vi "Adquisicion_6008.vi"() -> ()   [LabVIEW 2011]
uses:
  <vilib>/Utility/config.llb/Read Key (String).vi
  <vilib>/Utility/config.llb/Read Key (Double).vi
  <vilib>/Utility/config.llb/Write Key (String).vi
  <vilib>/Utility/config.llb/Write Key (Double).vi
  <vilib>/Utility/config.llb/NI_LVConfig.lvlib
  <vilib>/Analysis/NI_AALBase.lvlib
panel:
  out "Boolean 10":bool
  in  "Guardar":bool
  in  "Path2":bool
  in  "Datapath":bool
  in  "Path1":bool=TRUE
  in  "Tiempo":dbl
  in  "index 3":i32
  in  "index":i32
  out "reset3":bool
  out "reset2":bool
  out "reset":bool
  out "Time has Elapsed 2":bool caption="Time has Elapsed"
  out "Time has Elapsed":bool
  out "appended array":string[](array[string])
  in  "Tab Control 9":enum32{"Page 1", "Page 2", "Page 3"}(tab)
  in  "Tasa de Adquisicion":dbl=1000.0
  in  "CH8":string="CH8"
  in  "CH7":string="CH7"
  in  "CH6":string="CH6"
  in  "CH5":string="CH5"
  in  "CH4 2":string="CH4"
  in  "CH3":string="CH3"
  in  "CH2 2":string="CH2"
  in  "CH1":string="CH1"
  out "Voltaje":dbl
  out "Medida":dbl
  in  "m1":dbl
  in  "b1":dbl
  out "Voltaje":dbl
  in  "m2":dbl
  in  "b2":dbl
  out "Medida":dbl
  in  "m3":dbl
  in  "m4":dbl
  in  "b3":dbl
  in  "b4":dbl
  out "Voltaje":dbl
  out "Voltaje":dbl
  out "Medida":dbl
  out "Medida":dbl
  out "Medida":dbl
  in  "b5":dbl
  in  "m5":dbl
  out "Voltaje":dbl
  out "Medida":dbl
  in  "m6":dbl
  in  "b6":dbl
  out "Voltaje":dbl
  out "Medida":dbl
  in  "m7":dbl
  in  "b7":dbl
  out "Voltaje":dbl
  out "Voltaje":dbl
  in  "b8":dbl
  in  "m8":dbl
  out "Medida":dbl
  out "CH1":string
  out "CH2":string
  out "CH3":string
  out "CH4":string
  out "CH5":string
  out "CH6":string
  out "CH7":string
  out "CH8":string
  in  "Boolean":bool=TRUE
  in  "Boolean 2":bool=TRUE
  in  "Boolean 3":bool=TRUE
  in  "Boolean 4":bool=TRUE
  in  "Boolean 6":bool=TRUE
  in  "Boolean 5":bool=TRUE
  in  "Boolean 7":bool=TRUE
  in  "Boolean 8":bool=TRUE
  in  "Numero de Muestras":i32=1
  in  "file path":path=path "C:/Users/Zulueta/Documents/Pasantia/Mediciones"
  out "Tiempo":dbl caption="Elapsed Time (s)"
  in  "Iniciar":bool
  out "Boolean 9":bool
  in  "reset 2":bool caption="reset"
  out "q'":bool
  out "Tiempo":dbl caption="Elapsed Time (s)"
  in  "file path 2":path=path "C:/Users/Zulueta/Documents/Pasantia/Mediciones_Tiempo"
  out "Tiempo":dbl caption="Elapsed Time (s)"
  out "q2'":bool
  in  "?":bool
  in  "file path 3":path=path "C:/Users/Zulueta/Documents/Pasantia/Mediciones_Promedio"
  in  "Tiempo \nde adquisición":enum32{"Segundos", "Minutos", "Horas"}(tab) caption="Tiempo de adquisición"
  in  "?":dbl
  in  "?":dbl
  in  "?":dbl
  in  "stop":bool
  in  "Guardar Configuracion":bool
  out "Waveform Chart 10":dbl(graph)
  out "Waveform Chart 9":dbl(graph)
  out "Waveform Chart 8":dbl(graph)
  out "Waveform Chart 7":dbl(graph)
  out "Waveform Chart 6":dbl(graph)
  out "Waveform Chart 5":dbl(graph)
  out "Waveform Chart 4":dbl(graph)
  out "Waveform Chart 3":dbl(graph)
  out "CH1":string
  out "CH2":string
  out "CH3":string
  out "CH4":string
  out "CH5":string
  out "CH6":string
  out "CH7":string
  out "CH8":string
  in  "Boolean 18":bool=TRUE
  in  "Boolean 19":bool=TRUE
  in  "Boolean 20":bool=TRUE
  in  "Boolean 21":bool=TRUE
  in  "Boolean 22":bool=TRUE
  in  "Boolean 23":bool=TRUE
  in  "Boolean 24":bool=TRUE
  in  "Boolean 25":bool=TRUE
  out "Waveform Chart":cluster{dbl, dbl, dbl, dbl, dbl, dbl, dbl, dbl}(graph)
  out "Time":dbl
  # "On/Off"
  # "Pendiente"
  # "Medida"
  # "Offset"
  # "Voltaje"
  # "Aquirir muestras por solicitud"
  # "Adquirir muestras por tiempo definido"
  # "Adquirir promedio de cada canal en un tiempo T"
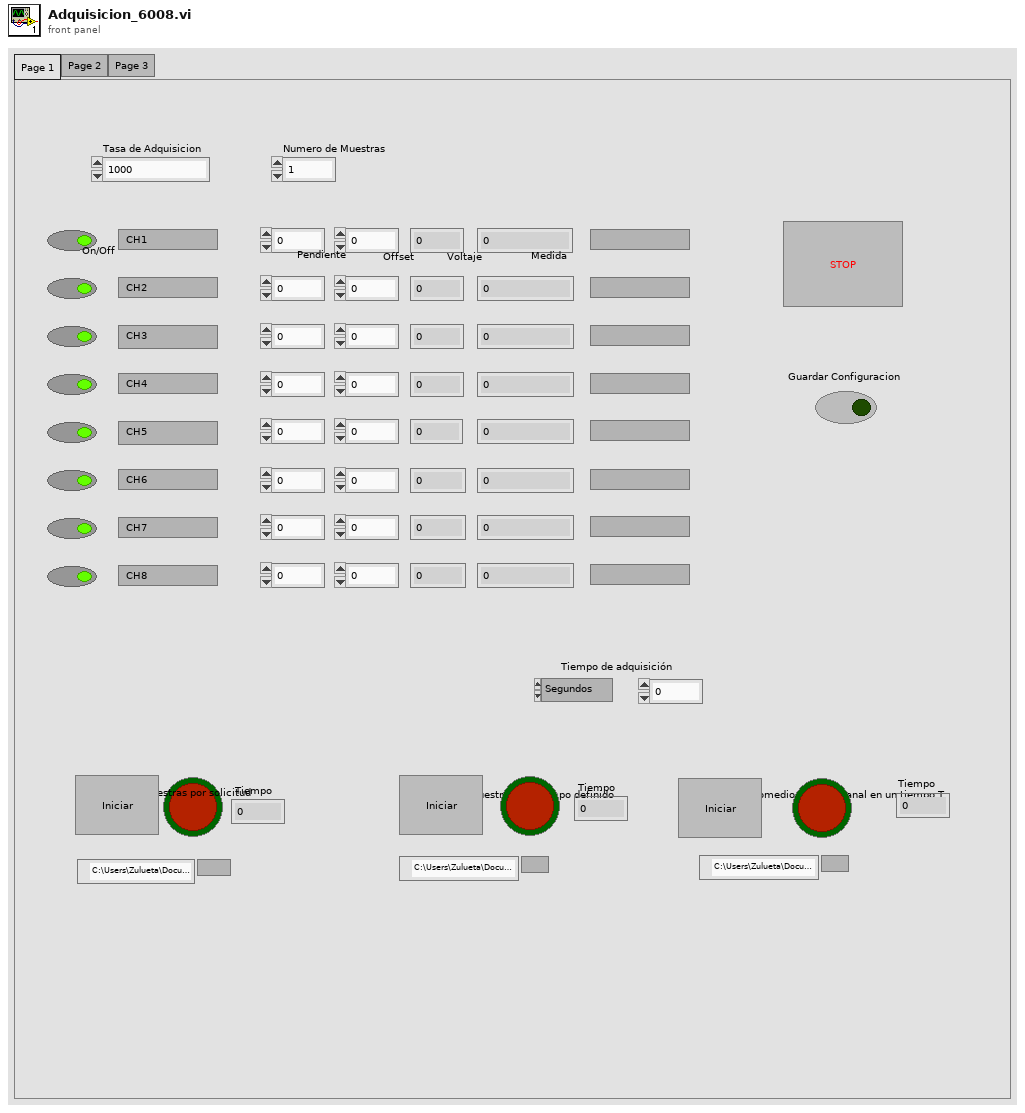
[diagram p1: front panel]
types:
  T1 = enum16{"big-endian, network order", "native, host order", "little-endian"}
  T2 = enum16{"open", "open or create", "create or replace", "create", "open (read-only)"}
  T3 = typedef "NI_LVConfig.lvlib/Config Data RefNum.ctl" = refnum<k1>
  T4 = cluster{"mean":dbl, "mean":dbl, "mean":dbl, "mean":dbl, "mean":dbl, "mean":dbl, "mean":dbl, "mean":dbl}
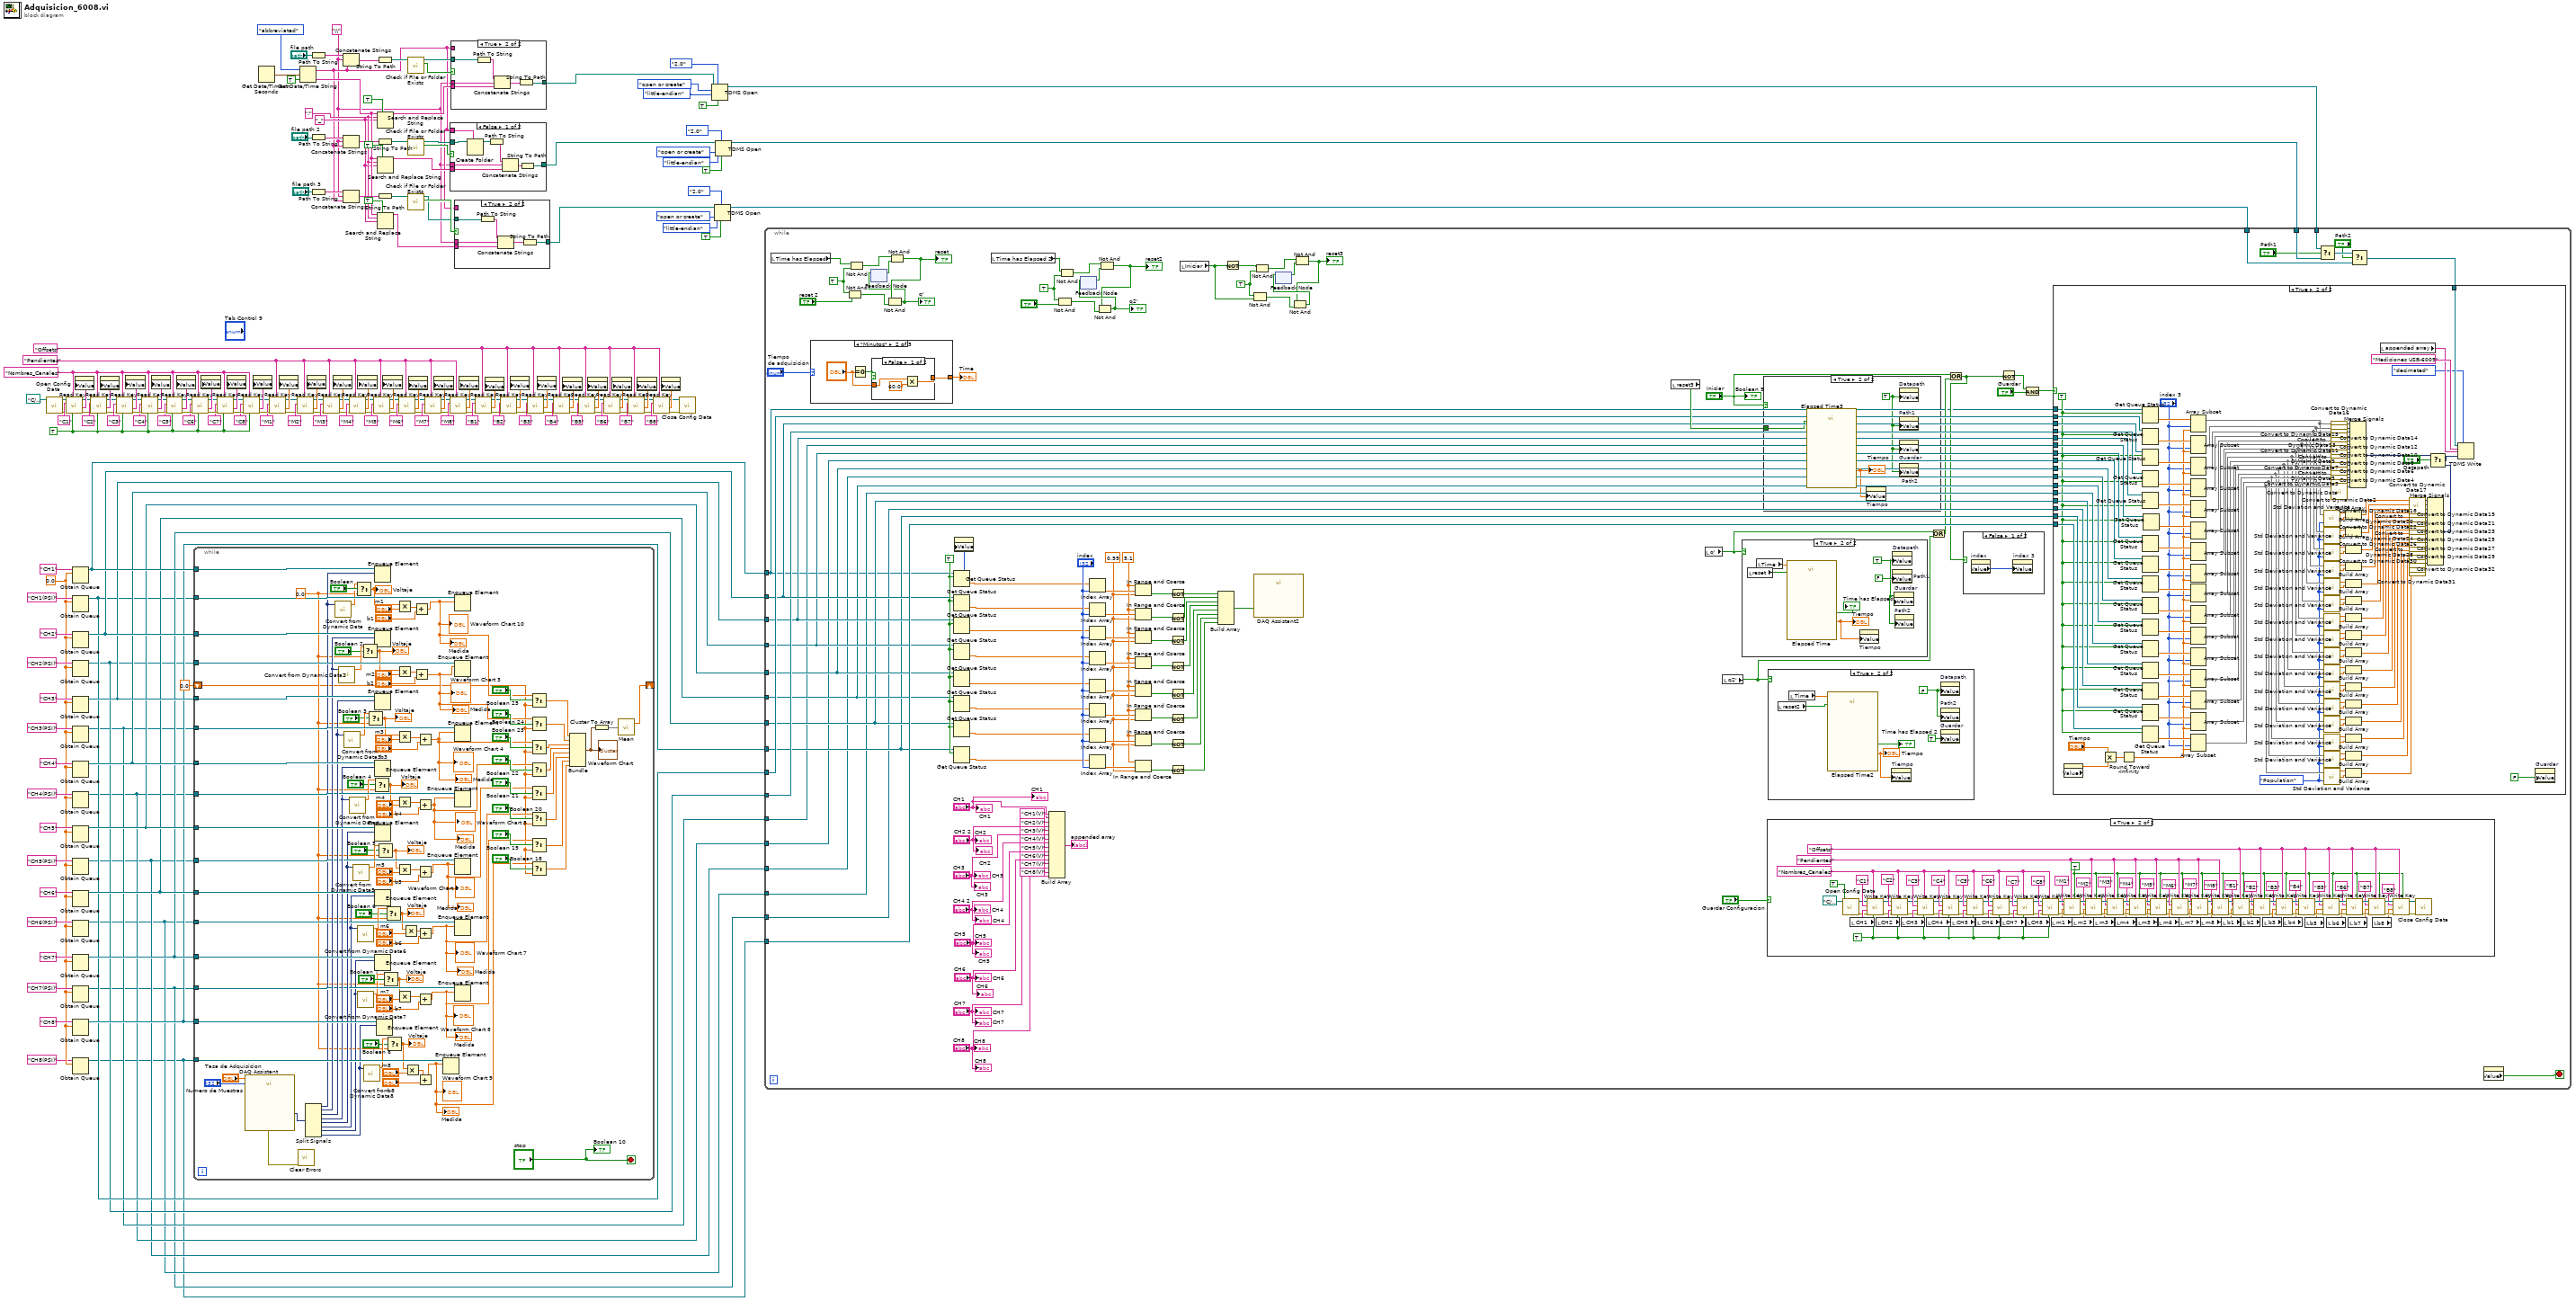
[diagram p0: block diagram]
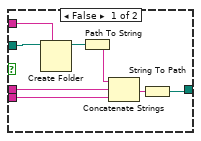
[diagram p2: hidden frame]
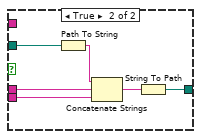
[diagram p3: hidden frame]
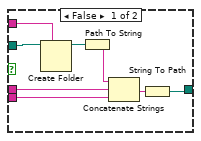
[diagram p4: hidden frame]
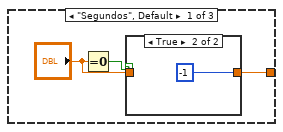
[diagram p11: hidden frame]
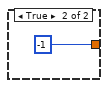
[diagram p13: hidden frame]
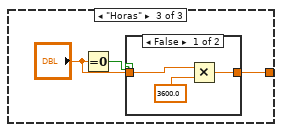
[diagram p14: hidden frame]
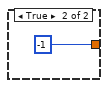
[diagram p15: hidden frame]
diagram:
  w25 = "_" ("replace string (\"\")")
  w26 = ":" ("search string")
  w9 = "\\" ("string")
  w71 = 0.0
  w88 = "Offsets" ("section")
  w121 = "Pendientes" ("section")
  w153 = TRUE ("read raw string? (F)")
  w154 = "Nombres_Canales" ("section")
  n1 = call <vilib>:"Open Config Data.vi"("configuration file path"=path "C:/Users/Zulueta/Documents/Pasantia/Configuracion") -> ("error out"=w183:errorcluster, "refnum"=w184:T3)  [unwired: 8 in, 1 out]
  n2 = call-poly <vilib>:"Read Key.vi"("read raw string? (F)"=w153, "section"=w154, "error in (no error)"=w183, "key"="C1", "refnum"=w184) -> ("error out"=w179:errorcluster, "value"=w186:string, "refnum out"=w180:T3)  [unwired: 3 in, 1 out]
  n3 = Obtain Queue(name (unnamed)="CH1", element data type=w71) -> (queue out=w69:refnum<queue>)  [unwired: 3 in, 2 out]
  n4 = Obtain Queue(name (unnamed)="CH1(PSI)", element data type=w71) -> (queue out=w59:refnum<queue>)  [unwired: 3 in, 2 out]
  n5 = Obtain Queue(name (unnamed)="CH2", element data type=w71) -> (queue out=w68:refnum<queue>)  [unwired: 3 in, 2 out]
  n6 = Obtain Queue(name (unnamed)="CH2(PSI)", element data type=w71) -> (queue out=w58:refnum<queue>)  [unwired: 3 in, 2 out]
  n7 = Obtain Queue(name (unnamed)="CH3", element data type=w71) -> (queue out=w67:refnum<queue>)  [unwired: 3 in, 2 out]
  n8 = Obtain Queue(name (unnamed)="CH3(PSI)", element data type=w71) -> (queue out=w57:refnum<queue>)  [unwired: 3 in, 2 out]
  n9 = Obtain Queue(name (unnamed)="CH4", element data type=w71) -> (queue out=w66:refnum<queue>)  [unwired: 3 in, 2 out]
  n10 = Obtain Queue(name (unnamed)="CH4(PSI)", element data type=w71) -> (queue out=w56:refnum<queue>)  [unwired: 3 in, 2 out]
  n11 = Obtain Queue(name (unnamed)="CH5", element data type=w71) -> (queue out=w65:refnum<queue>)  [unwired: 3 in, 2 out]
  n12 = Obtain Queue(name (unnamed)="CH5(PSI)", element data type=w71) -> (queue out=w55:refnum<queue>)  [unwired: 3 in, 2 out]
  n13 = Obtain Queue(name (unnamed)="CH6", element data type=w71) -> (queue out=w64:refnum<queue>)  [unwired: 3 in, 2 out]
  n14 = Obtain Queue(name (unnamed)="CH6(PSI)", element data type=w71) -> (queue out=w54:refnum<queue>)  [unwired: 3 in, 2 out]
  n15 = Obtain Queue(name (unnamed)="CH7", element data type=w71) -> (queue out=w63:refnum<queue>)  [unwired: 3 in, 2 out]
  n16 = Obtain Queue(name (unnamed)="CH7(PSI)", element data type=w71) -> (queue out=w53:refnum<queue>)  [unwired: 3 in, 2 out]
  n17 = Obtain Queue(name (unnamed)="CH8", element data type=w71) -> (queue out=w62:refnum<queue>)  [unwired: 3 in, 2 out]
  n18 = Obtain Queue(name (unnamed)="CH8(PSI)", element data type=w71) -> (queue out=w52:refnum<queue>)  [unwired: 3 in, 2 out]
  n19 = property on="CH1" class="Str"("Value"=w186) -> ()  [unwired: 2 in, 2 out]
  n20 = call-poly <vilib>:"Read Key.vi"("read raw string? (F)"=w153, "section"=w154, "error in (no error)"=w179, "key"="C2", "refnum"=w180) -> ("error out"=w176:errorcluster, "value"=w181:string, "refnum out"=w175:T3)  [unwired: 3 in, 1 out]
  n21 = property on="CH2 2" class="Str"("Value"=w181) -> ()  [unwired: 2 in, 2 out]
  n22 = call-poly <vilib>:"Read Key.vi"("read raw string? (F)"=w153, "section"=w154, "error in (no error)"=w176, "key"="C3", "refnum"=w175) -> ("error out"=w172:errorcluster, "value"=w178:string, "refnum out"=w173:T3)  [unwired: 3 in, 1 out]
  n23 = property on="CH3" class="Str"("Value"=w178) -> ()  [unwired: 2 in, 2 out]
  n24 = call-poly <vilib>:"Read Key.vi"("read raw string? (F)"=w153, "section"=w154, "error in (no error)"=w172, "key"="C4", "refnum"=w173) -> ("error out"=w169:errorcluster, "value"=w174:string, "refnum out"=w170:T3)  [unwired: 3 in, 1 out]
  n25 = property on="CH4 2" class="Str"("Value"=w174) -> ()  [unwired: 2 in, 2 out]
  n26 = call-poly <vilib>:"Read Key.vi"("read raw string? (F)"=w153, "section"=w154, "error in (no error)"=w169, "key"="C5", "refnum"=w170) -> ("error out"=w164:errorcluster, "value"=w167:string, "refnum out"=w165:T3)  [unwired: 3 in, 1 out]
  n27 = property on="CH5" class="Str"("Value"=w167) -> ()  [unwired: 2 in, 2 out]
  n28 = call-poly <vilib>:"Read Key.vi"("read raw string? (F)"=w153, "section"=w154, "error in (no error)"=w164, "key"="C6", "refnum"=w165) -> ("error out"=w161:errorcluster, "value"=w166:string, "refnum out"=w162:T3)  [unwired: 3 in, 1 out]
  n29 = while {
    tunnel: w69 -> [w197]
    tunnel: w68 -> [w293]
    tunnel: w67 -> [w292]
    tunnel: w66 -> [w291]
    tunnel: w65 -> [w290]
    tunnel: w64 -> [w289]
    tunnel: w63 -> [w288]
    tunnel: w62 -> [w287]
    tunnel: w59 -> [w283]
    tunnel: w58 -> [w278]
    tunnel: w57 -> [w277]
    tunnel: w56 -> [w272]
    tunnel: w54 -> [w262]
    tunnel: w55 -> [w267]
    tunnel: w53 -> [w261]
    tunnel: w52 -> [w260]
    shift-right: [w194] -> _
    shift-left: 0.0 ("mean") -> [w193]
    stop <- "stop" stop-if-true
    w223 = 0.0 ("f")
    n30 = call "DAQ Assistant"("rate"="Tasa de Adquisicion", "number of samples"="Numero de Muestras") -> ("data"=w188:dynamicdata, "error out"=w191:errorcluster)  [unwired: 14 in, 2 out]
    n31 = call <vilib>:"Clear Errors.vi"("error in (no error)"=w191) -> ()  [unwired: 6 in, 1 out]
    n32 = Split Signals(w188) -> (w246:dynamicdata, w281:dynamicdata, w276:dynamicdata, w271:dynamicdata, w266:dynamicdata, w259:dynamicdata, w255:dynamicdata, w251:dynamicdata)  [unwired: 8 in]
    n33 = call "Convert from Dynamic Data"("Dynamic Data Type"=w246) -> ("Scalar"=w235:dbl)  [unwired: 3 in]
    n34 = call "Convert from Dynamic Data2"("Dynamic Data Type"=w281) -> ("Scalar"=w245:dbl)  [unwired: 3 in]
    n35 = call "Convert from Dynamic Data3"("Dynamic Data Type"=w276) -> ("Scalar"=w243:dbl)  [unwired: 3 in]
    n36 = call "Convert from Dynamic Data4"("Dynamic Data Type"=w271) -> ("Scalar"=w241:dbl)  [unwired: 3 in]
    n37 = call "Convert from Dynamic Data5"("Dynamic Data Type"=w266) -> ("Scalar"=w239:dbl)  [unwired: 3 in]
    n38 = Select(t=w235, s="Boolean", f=w223) -> (s? t:f=w234:dbl)
    "Voltaje" <- w234
    n39 = call "Convert from Dynamic Data6"("Dynamic Data Type"=w259) -> ("Scalar"=w237:dbl)  [unwired: 3 in]
    n40 = call "Convert from Dynamic Data7"("Dynamic Data Type"=w255) -> ("Scalar"=w227:dbl)  [unwired: 3 in]
    n41 = Select(t=w245, s="Boolean 2", f=w223) -> (s? t:f=w233:dbl)
    "Voltaje" <- w233
    n42 = call "Convert from Dynamic Data8"("Dynamic Data Type"=w251) -> ("Scalar"=w225:dbl)  [unwired: 3 in]
    n43 = Select(t=w243, s="Boolean 3", f=w223) -> (s? t:f=w232:dbl)
    "Voltaje" <- w232
    n44 = Select(t=w241, s="Boolean 4", f=w223) -> (s? t:f=w231:dbl)
    "Voltaje" <- w231
    n45 = Enqueue Element(queue=w197, element=w246) -> ()  [unwired: 2 in, 3 out]
    n46 = Enqueue Element(queue=w293, element=w281) -> ()  [unwired: 2 in, 3 out]
    n47 = Enqueue Element(queue=w292, element=w276) -> ()  [unwired: 2 in, 3 out]
    n48 = Enqueue Element(queue=w291, element=w271) -> ()  [unwired: 2 in, 3 out]
    n49 = Enqueue Element(queue=w290, element=w266) -> ()  [unwired: 2 in, 3 out]
    n50 = Enqueue Element(queue=w289, element=w259) -> ()  [unwired: 2 in, 3 out]
    n51 = Enqueue Element(queue=w288, element=w255) -> ()  [unwired: 2 in, 3 out]
    n52 = Enqueue Element(queue=w287, element=w251) -> ()  [unwired: 2 in, 3 out]
    n53 = Select(t=w239, s="Boolean 5", f=w223) -> (s? t:f=w230:dbl)
    "Voltaje" <- w230
    n54 = Select(t=w227, s="Boolean 7", f=w223) -> (s? t:f=w226:dbl)
    "Voltaje" <- w226
    n55 = Select(t=w237, s="Boolean 6", f=w223) -> (s? t:f=w229:dbl)
    "Voltaje" <- w229
    n56 = Select(t=w225, s="Boolean 8", f=w223) -> (s? t:f=w224:dbl)
    "Voltaje" <- w224
    n57 = Multiply(x=w234, y="m1") -> (x*y=w285:dbl)
    n58 = Multiply(x=w233, y="m2") -> (x*y=w280:dbl)
    n59 = Multiply(x=w232, y="m3") -> (x*y=w274:dbl)
    n60 = Multiply(x=w231, y="m4") -> (x*y=w269:dbl)
    n61 = Multiply(x=w230, y="m5") -> (x*y=w264:dbl)
    n62 = Multiply(x=w226, y="m7") -> (x*y=w253:dbl)
    n63 = Multiply(x=w229, y="m6") -> (x*y=w257:dbl)
    n64 = Multiply(x=w224, y="m8") -> (x*y=w249:dbl)
    n65 = Add(x=w285, y="b1") -> (x+y=w213:dbl)
    "Waveform Chart 10" <- w213
    "Medida" <- w213
    n66 = Add(x=w280, y="b2") -> (x+y=w212:dbl)
    "Waveform Chart 3" <- w212
    "Medida" <- w212
    n67 = Add(x=w274, y="b3") -> (x+y=w211:dbl)
    "Waveform Chart 4" <- w211
    "Medida" <- w211
    n68 = Add(x=w269, y="b4") -> (x+y=w210:dbl)
    "Waveform Chart 5" <- w210
    "Medida" <- w210
    n69 = Add(x=w264, y="b5") -> (x+y=w209:dbl)
    "Waveform Chart 6" <- w209
    "Medida" <- w209
    n70 = Add(x=w257, y="b6") -> (x+y=w208:dbl)
    "Waveform Chart 7" <- w208
    "Medida" <- w208
    n71 = Add(x=w253, y="b7") -> (x+y=w207:dbl)
    "Waveform Chart 8" <- w207
    "Medida" <- w207
    n72 = Add(x=w249, y="b8") -> (x+y=w206:dbl)
    "Waveform Chart 9" <- w206
    "Medida" <- w206
    n73 = Enqueue Element(queue=w260, element=w206) -> ()  [unwired: 2 in, 3 out]
    n74 = Enqueue Element(queue=w283, element=w213) -> ()  [unwired: 2 in, 3 out]
    n75 = Enqueue Element(queue=w278, element=w212) -> ()  [unwired: 2 in, 3 out]
    n76 = Enqueue Element(queue=w277, element=w211) -> ()  [unwired: 2 in, 3 out]
    n77 = Enqueue Element(queue=w272, element=w210) -> ()  [unwired: 2 in, 3 out]
    n78 = Enqueue Element(queue=w267, element=w209) -> ()  [unwired: 2 in, 3 out]
    n79 = Enqueue Element(queue=w262, element=w208) -> ()  [unwired: 2 in, 3 out]
    n80 = Enqueue Element(queue=w261, element=w207) -> ()  [unwired: 2 in, 3 out]
    n81 = Select(t=w213, s="Boolean 25", f=w193) -> (s? t:f=w205:dbl)
    n82 = Select(t=w212, s="Boolean 24", f=w193) -> (s? t:f=w204:dbl)
    n83 = Select(t=w211, s="Boolean 23", f=w193) -> (s? t:f=w203:dbl)
    n84 = Select(t=w210, s="Boolean 22", f=w193) -> (s? t:f=w202:dbl)
    n85 = Select(t=w209, s="Boolean 21", f=w193) -> (s? t:f=w201:dbl)
    n86 = Select(t=w208, s="Boolean 20", f=w193) -> (s? t:f=w200:dbl)
    n87 = Select(t=w207, s="Boolean 19", f=w193) -> (s? t:f=w199:dbl)
    n88 = Select(t=w206, s="Boolean 18", f=w193) -> (s? t:f=w198:dbl)
    n89 = Bundle("mean"=w205, "mean"=w204, "mean"=w203, "mean"=w202, "mean"=w201, "mean"=w200, "mean"=w199, "mean"=w198) -> (w196:T4)  [unwired: 1 in]
    "Waveform Chart" <- w196
    n90 = Cluster To Array(cluster=w196) -> (array=w195:dbl[])
    n91 = call <vilib>:"Mean.vi"("X"=w195) -> ("mean"=w194:dbl)  [unwired: 1 out]
    "Boolean 10" <- "stop"
  }
  n92 = property on="CH6" class="Str"("Value"=w166) -> ()  [unwired: 2 in, 2 out]
  n93 = call-poly <vilib>:"Read Key.vi"("read raw string? (F)"=w153, "section"=w154, "error in (no error)"=w161, "key"="C7", "refnum"=w162) -> ("error out"=w156:errorcluster, "value"=w160:string, "refnum out"=w157:T3)  [unwired: 3 in, 1 out]
  n94 = property on="CH7" class="Str"("Value"=w160) -> ()  [unwired: 2 in, 2 out]
  n95 = call-poly <vilib>:"Read Key.vi"("read raw string? (F)"=w153, "section"=w154, "error in (no error)"=w156, "key"="C8", "refnum"=w157) -> ("error out"=w151:errorcluster, "value"=w158:string, "refnum out"=w152:T3)  [unwired: 3 in, 1 out]
  n96 = property on="CH8" class="Str"("Value"=w158) -> ()  [unwired: 2 in, 2 out]
  n97 = Get Date/Time In Seconds() -> (seconds since 1Jan1904=w36:timestamp)
  n98 = call-poly <vilib>:"Read Key.vi"("section"=w121, "error in (no error)"=w151, "key"="M1", "refnum"=w152) -> ("error out"=w146:errorcluster, "value"=w150:dbl, "refnum out"=w147:T3)  [unwired: 4 in, 1 out]
  n99 = property on="m1" class="DigNum (strict)"("Value"=w150) -> ()  [unwired: 2 in, 2 out]
  n100 = call-poly <vilib>:"Read Key.vi"("section"=w121, "error in (no error)"=w146, "key"="M2", "refnum"=w147) -> ("error out"=w142:errorcluster, "value"=w145:dbl, "refnum out"=w143:T3)  [unwired: 4 in, 1 out]
  n101 = Get Date/Time String(date format (0)=enum16{"short", "long", "abbreviated"}."abbreviated", seconds (now)=w36, want seconds? (F)=TRUE) -> (date string=w10:string, time string=w27:string)
  n102 = property on="m2" class="DigNum (strict)"("Value"=w145) -> ()  [unwired: 2 in, 2 out]
  n103 = Path To String(path="file path") -> (string=w40:string)
  n104 = Path To String(path="file path 2") -> (string=w32:string)
  n105 = Path To String(path="file path 3") -> (string=w29:string)
  n106 = call-poly <vilib>:"Read Key.vi"("section"=w121, "error in (no error)"=w142, "key"="M3", "refnum"=w143) -> ("error out"=w139:errorcluster, "value"=w141:dbl, "refnum out"=w138:T3)  [unwired: 4 in, 1 out]
  n107 = property on="m3" class="DigNum (strict)"("Value"=w141) -> ()  [unwired: 2 in, 2 out]
  n108 = Concatenate Strings(w40, w9, w10) -> (w38:string)
  n109 = Concatenate Strings(w32, w9, w10) -> (w33:string)
  n110 = Concatenate Strings(w29, w9, w10) -> (w28:string)
  n111 = call-poly <vilib>:"Read Key.vi"("section"=w121, "error in (no error)"=w139, "key"="M4", "refnum"=w138) -> ("error out"=w135:errorcluster, "value"=w137:dbl, "refnum out"=w134:T3)  [unwired: 4 in, 1 out]
  n112 = property on="m4" class="DigNum (strict)"("Value"=w137) -> ()  [unwired: 2 in, 2 out]
  n113 = call-poly <vilib>:"Read Key.vi"("section"=w121, "error in (no error)"=w135, "key"="M5", "refnum"=w134) -> ("error out"=w131:errorcluster, "value"=w133:dbl, "refnum out"=w130:T3)  [unwired: 4 in, 1 out]
  n114 = String To Path(string=w38) -> (path=w39:path)
  n115 = String To Path(string=w33) -> (path=w34:path)
  n116 = String To Path(string=w28) -> (path=w24:path)
  n117 = Search and Replace String(replace all?=TRUE ("replace all? (F)"), input string=w27, search string=w26, replace string=w25) -> (result string=w19:string)  [unwired: 4 in, 3 out]
  n118 = Search and Replace String(replace all?=TRUE ("replace all? (F)"), input string=w27, search string=w26, replace string=w25) -> (result string=w13:string)  [unwired: 4 in, 3 out]
  n119 = Search and Replace String(replace all?=TRUE ("replace all? (F)"), input string=w27, search string=w26, replace string=w25) -> (result string=w8:string)  [unwired: 4 in, 3 out]
  n120 = property on="m5" class="DigNum (strict)"("Value"=w133) -> ()  [unwired: 2 in, 2 out]
  n121 = call-poly <vilib>:"Read Key.vi"("section"=w121, "error in (no error)"=w131, "key"="M6", "refnum"=w130) -> ("error out"=w126:errorcluster, "value"=w129:dbl, "refnum out"=w127:T3)  [unwired: 4 in, 1 out]
  n122 = call <vilib>:"Check if File or Folder Exists.vi"("path"=w39) -> ("file or folder exists?"=w17:bool, "dup path"=w20:path)  [unwired: 8 in, 1 out]
  n123 = call <vilib>:"Check if File or Folder Exists.vi"("path"=w34) -> ("file or folder exists?"=w16:bool, "dup path"=w15:path)  [unwired: 8 in, 1 out]
  n124 = call <vilib>:"Check if File or Folder Exists.vi"("path"=w24) -> ("file or folder exists?"=w12:bool, "dup path"=w11:path)  [unwired: 8 in, 1 out]
  n125 = property on="m6" class="DigNum (strict)"("Value"=w129) -> ()  [unwired: 2 in, 2 out]
  n126 = call-poly <vilib>:"Read Key.vi"("section"=w121, "error in (no error)"=w126, "key"="M7", "refnum"=w127) -> ("error out"=w123:errorcluster, "value"=w125:dbl, "refnum out"=w122:T3)  [unwired: 4 in, 1 out]
  n127 = property on="m7" class="DigNum (strict)"("Value"=w125) -> ()  [unwired: 2 in, 2 out]
  n128 = case shown="False" w16 {
    tunnel: w15 -> [w300 w307]
    tunnel: w9 -> [w298 w304]
    tunnel: w13 -> [w297 w303]
    tunnel: [w295 w302] -> w14
    tunnel: w10 -> [w294 _]
    frame False {
      n129 = Create Folder(prompt (Create Folder)=w294, path (use dialog)=w300) -> (created path=w301:path)  [unwired: 1 in, 2 out]
      n130 = Path To String(path=w301) -> (string=w299:string)
      n131 = Concatenate Strings(w299, w298, w297) -> (w296:string)
      n132 = String To Path(string=w296) -> (path=w295:path)
    }
    frame True {
      n133 = Path To String(path=w307) -> (string=w305:string)
      n134 = Concatenate Strings(w305, w304, w303) -> (w306:string)
      n135 = String To Path(string=w306) -> (path=w302:path)
    }
  }
  n136 = call-poly <vilib>:"Read Key.vi"("section"=w121, "error in (no error)"=w123, "key"="M8", "refnum"=w122) -> ("error out"=w118:errorcluster, "value"=w120:dbl, "refnum out"=w117:T3)  [unwired: 4 in, 1 out]
  n137 = case shown="True" w17 {
    tunnel: w20 -> [w314 w321]
    tunnel: w9 -> [w312 w318]
    tunnel: w19 -> [w311 w317]
    tunnel: [w309 w316] -> w18
    tunnel: w10 -> [w308 _]
    frame False {
      n138 = Create Folder(prompt (Create Folder)=w308, path (use dialog)=w314) -> (created path=w315:path)  [unwired: 1 in, 2 out]
      n139 = Path To String(path=w315) -> (string=w313:string)
      n140 = Concatenate Strings(w313, w312, w311) -> (w310:string)
      n141 = String To Path(string=w310) -> (path=w309:path)
    }
    frame True {
      n142 = Path To String(path=w321) -> (string=w319:string)
      n143 = Concatenate Strings(w319, w318, w317) -> (w320:string)
      n144 = String To Path(string=w320) -> (path=w316:path)
    }
  }
  n145 = case shown="True" w12 {
    tunnel: w11 -> [w328 w335]
    tunnel: w9 -> [w326 w332]
    tunnel: w8 -> [w325 w331]
    tunnel: [w323 w330] -> w7
    tunnel: w10 -> [w322 _]
    frame False {
      n146 = Create Folder(prompt (Create Folder)=w322, path (use dialog)=w328) -> (created path=w329:path)  [unwired: 1 in, 2 out]
      n147 = Path To String(path=w329) -> (string=w327:string)
      n148 = Concatenate Strings(w327, w326, w325) -> (w324:string)
      n149 = String To Path(string=w324) -> (path=w323:path)
    }
    frame True {
      n150 = Path To String(path=w335) -> (string=w333:string)
      n151 = Concatenate Strings(w333, w332, w331) -> (w334:string)
      n152 = String To Path(string=w334) -> (path=w330:path)
    }
  }
  n153 = property on="m8" class="DigNum (strict)"("Value"=w120) -> ()  [unwired: 2 in, 2 out]
  n154 = call-poly <vilib>:"Read Key.vi"("section"=w88, "error in (no error)"=w118, "key"="B1", "refnum"=w117) -> ("error out"=w114:errorcluster, "value"=w116:dbl, "refnum out"=w113:T3)  [unwired: 4 in, 1 out]
  n155 = property on="b1" class="DigNum (strict)"("Value"=w116) -> ()  [unwired: 2 in, 2 out]
  n156 = call-poly <vilib>:"Read Key.vi"("section"=w88, "error in (no error)"=w114, "key"="B2", "refnum"=w113) -> ("error out"=w110:errorcluster, "value"=w112:dbl, "refnum out"=w109:T3)  [unwired: 4 in, 1 out]
  n157 = property on="b2" class="DigNum (strict)"("Value"=w112) -> ()  [unwired: 2 in, 2 out]
  n158 = call-poly <vilib>:"Read Key.vi"("section"=w88, "error in (no error)"=w110, "key"="B3", "refnum"=w109) -> ("error out"=w106:errorcluster, "value"=w108:dbl, "refnum out"=w105:T3)  [unwired: 4 in, 1 out]
  n159 = property on="b3" class="DigNum (strict)"("Value"=w108) -> ()  [unwired: 2 in, 2 out]
  n160 = call-poly <vilib>:"Read Key.vi"("section"=w88, "error in (no error)"=w106, "key"="B4", "refnum"=w105) -> ("error out"=w101:errorcluster, "value"=w104:dbl, "refnum out"=w102:T3)  [unwired: 4 in, 1 out]
  n161 = property on="b4" class="DigNum (strict)"("Value"=w104) -> ()  [unwired: 2 in, 2 out]
  n162 = call-poly <vilib>:"Read Key.vi"("section"=w88, "error in (no error)"=w101, "key"="B5", "refnum"=w102) -> ("error out"=w98:errorcluster, "value"=w100:dbl, "refnum out"=w97:T3)  [unwired: 4 in, 1 out]
  n163 = property on="b5" class="DigNum (strict)"("Value"=w100) -> ()  [unwired: 2 in, 2 out]
  n164 = call-poly <vilib>:"Read Key.vi"("section"=w88, "error in (no error)"=w98, "key"="B6", "refnum"=w97) -> ("error out"=w93:errorcluster, "value"=w96:dbl, "refnum out"=w94:T3)  [unwired: 4 in, 1 out]
  n165 = property on="b6" class="DigNum (strict)"("Value"=w96) -> ()  [unwired: 2 in, 2 out]
  n166 = call-poly <vilib>:"Read Key.vi"("section"=w88, "error in (no error)"=w93, "key"="B7", "refnum"=w94) -> ("error out"=w89:errorcluster, "value"=w92:dbl, "refnum out"=w90:T3)  [unwired: 4 in, 1 out]
  n167 = property on="b7" class="DigNum (strict)"("Value"=w92) -> ()  [unwired: 2 in, 2 out]
  n168 = call-poly <vilib>:"Read Key.vi"("section"=w88, "error in (no error)"=w89, "key"="B8", "refnum"=w90) -> ("error out"=w60:errorcluster, "value"=w87:dbl, "refnum out"=w61:T3)  [unwired: 4 in, 1 out]
  n169 = property on="b8" class="DigNum (strict)"("Value"=w87) -> ()  [unwired: 2 in, 2 out]
  n170 = call <vilib>:"Close Config Data.vi"("error in (no error)"=w60, "refnum"=w61) -> ()  [unwired: 8 in, 2 out]
  n171 = TDMS Open(6:TRUE ("disable buffering? (T)"), 7:enum16{"1.0", "2.0"}."2.0" ("file format version (2.0)"), 9:T1."little-endian" ("byte order (2:little-endian)"), 10:T2."open or create" ("operation (0:open)"), 11:w18) -> (3:w6:refnum<k34>)  [unwired: 1 in, 1 out]
  n172 = TDMS Open(6:TRUE ("disable buffering? (T)"), 7:enum16{"1.0", "2.0"}."2.0" ("file format version (2.0)"), 9:T1."little-endian" ("byte order (2:little-endian)"), 10:T2."open or create" ("operation (0:open)"), 11:w7) -> (3:w4:refnum<k34>)  [unwired: 1 in, 1 out]
  n173 = TDMS Open(6:TRUE ("disable buffering? (T)"), 7:enum16{"1.0", "2.0"}."2.0" ("file format version (2.0)"), 9:T1."little-endian" ("byte order (2:little-endian)"), 10:T2."open or create" ("operation (0:open)"), 11:w14) -> (3:w5:refnum<k34>)  [unwired: 1 in, 1 out]
  n174 = while {
    tunnel: w69 -> [w346]
    tunnel: w68 -> [w398]
    tunnel: w67 -> [w396]
    tunnel: w66 -> [w395]
    tunnel: w65 -> [w394]
    tunnel: w64 -> [w393]
    tunnel: w63 -> [w392]
    tunnel: w62 -> [w391]
    tunnel: w59 -> [w399]
    tunnel: w58 -> [w397]
    tunnel: w57 -> [w390]
    tunnel: w56 -> [w389]
    tunnel: w55 -> [w388]
    tunnel: w54 -> [w387]
    tunnel: w53 -> [w386]
    tunnel: w52 -> [w400]
    tunnel: w6 -> [w383]
    tunnel: w5 -> [w382]
    tunnel: w4 -> [w373]
    stop <- w337 stop-if-true
    w363 = 0.99 ("lower limit")
    w364 = 5.1 ("upper limit")
    w402 = TRUE ("return elements? (F)")
    w419 = TRUE ("y")
    w428 = TRUE ("y")
    w443 = TRUE ("y")
    n175 = local read "Time has Elapsed"() -> (w440:bool)
    n176 = case shown="\"Minutos\"" "Tiempo \nde adquisición" {
      tunnel: [w718 w721 w728] -> w449
      frame "Segundos", Default {
        n177 = Equal To 0?(x="?") -> (x = 0?=w717:bool)
        n178 = case shown="True" w717 {
          tunnel: [w719 -1] -> w718
          tunnel: "?" -> [w719 _]
          frame False {
          }
          frame True {
          }
        }
      }
      frame "Minutos" {
        n179 = Equal To 0?(x="?") -> (x = 0?=w723:bool)
        n180 = case shown="False" w723 {
          tunnel: [w724 -1] -> w721
          tunnel: "?" -> [w726 _]
          frame False {
            n181 = Multiply(x=w726, y=60.0) -> (x*y=w724:dbl)
          }
          frame True {
          }
        }
      }
      frame "Horas" {
        n182 = Equal To 0?(x="?") -> (x = 0?=w730:bool)
        n183 = case shown="False" w730 {
          tunnel: [w731 -1] -> w728
          tunnel: "?" -> [w733 _]
          frame False {
            n184 = Multiply(x=w733, y=3600.0) -> (x*y=w731:dbl)
          }
          frame True {
          }
        }
      }
    }
    "Time" <- w449
    n185 = Not And(1:"reset 2", 2:w443) -> (0:w446:bool)
    n186 = Not And(1:w443, 2:w440) -> (0:w441:bool)
    n187 = feedback #1() -> (w444:bool)  [unwired: 1 in]
    n188 = Not And(1:w444, 2:w441) -> (0:w447:bool)
    "reset" <- w447
    n189 = Not And(1:w446, 2:w447) -> (0:w445:bool)
    "q'" <- w445
    n190 = feedback-in #1(w445) -> ()
    n191 = Get Queue Status(queue=w398, return elements? (F)=w402) -> (elements=w344:dbl[])  [unwired: 1 in, 7 out]
    n192 = Get Queue Status(queue=w396, return elements? (F)=w402) -> (elements=w343:dbl[])  [unwired: 1 in, 7 out]
    n193 = Get Queue Status(queue=w395, return elements? (F)=w402) -> (elements=w342:dbl[])  [unwired: 1 in, 7 out]
    n194 = Get Queue Status(queue=w346, return elements? (F)=w402) -> (# elements in queue=w406:i32, elements=w345:dbl[])  [unwired: 1 in, 6 out]
    n195 = Get Queue Status(queue=w394, return elements? (F)=w402) -> (elements=w341:dbl[])  [unwired: 1 in, 7 out]
    n196 = Get Queue Status(queue=w393, return elements? (F)=w402) -> (elements=w339:dbl[])  [unwired: 1 in, 7 out]
    n197 = Get Queue Status(queue=w392, return elements? (F)=w402) -> (elements=w340:dbl[])  [unwired: 1 in, 7 out]
    n198 = Get Queue Status(queue=w391, return elements? (F)=w402) -> (elements=w338:dbl[])  [unwired: 1 in, 7 out]
    n199 = property on="index" class="DigNum (strict)"("Value"=w406) -> ()  [unwired: 2 in, 2 out]
    n200 = local read "Time has Elapsed 2"() -> (w424:bool)
    n201 = Build Array("CH1(V)" ("element"), "CH1", "CH2(V)" ("element"), "CH2 2", "CH3(V)" ("element"), "CH3", "CH4(V)" ("element"), "CH4 2", "CH5(V)" ("element"), "CH5", "CH6(V)" ("element"), "CH6", "CH7(V)" ("element"), "CH7", "CH8(V)" ("element"), "CH8") -> (→"appended array":string[])
    n202 = Not And(1:"?", 2:w428) -> (0:w431:bool)
    n203 = Not And(1:w428, 2:w424) -> (0:w427:bool)
    n204 = feedback #2() -> (w429:bool)  [unwired: 1 in]
    n205 = Index Array(array=w345, index="index") -> (element=w372:dbl)
    n206 = Index Array(array=w344, index="index") -> (element=w371:dbl)
    n207 = Index Array(array=w343, index="index") -> (element=w370:dbl)
    n208 = Index Array(array=w342, index="index") -> (element=w369:dbl)
    n209 = Index Array(array=w341, index="index") -> (element=w368:dbl)
    n210 = Index Array(array=w339, index="index") -> (element=w367:dbl)
    n211 = Index Array(array=w340, index="index") -> (element=w366:dbl)
    n212 = Index Array(array=w338, index="index") -> (element=w365:dbl)
    n213 = Not And(1:w429, 2:w427) -> (0:w426:bool)
    "reset2" <- w426
    n214 = Not And(1:w431, 2:w426) -> (0:w430:bool)
    "q2'" <- w430
    n215 = feedback-in #2(w430) -> ()
    n216 = In Range and Coerce(upper limit=w364, x=w372, lower limit=w363) -> (In Range?=w362:bool)  [unwired: 1 out]
    n217 = In Range and Coerce(upper limit=w364, x=w371, lower limit=w363) -> (In Range?=w361:bool)  [unwired: 1 out]
    n218 = In Range and Coerce(upper limit=w364, x=w370, lower limit=w363) -> (In Range?=w360:bool)  [unwired: 1 out]
    n219 = In Range and Coerce(upper limit=w364, x=w369, lower limit=w363) -> (In Range?=w359:bool)  [unwired: 1 out]
    n220 = In Range and Coerce(upper limit=w364, x=w368, lower limit=w363) -> (In Range?=w358:bool)  [unwired: 1 out]
    n221 = In Range and Coerce(upper limit=w364, x=w367, lower limit=w363) -> (In Range?=w357:bool)  [unwired: 1 out]
    n222 = In Range and Coerce(upper limit=w364, x=w366, lower limit=w363) -> (In Range?=w356:bool)  [unwired: 1 out]
    n223 = In Range and Coerce(upper limit=w364, x=w365, lower limit=w363) -> (In Range?=w355:bool)  [unwired: 1 out]
    n224 = Not(x=w362) -> (.not. x?=w354:bool)
    n225 = Not(x=w361) -> (.not. x?=w353:bool)
    n226 = Not(x=w360) -> (.not. x?=w352:bool)
    n227 = Not(x=w359) -> (.not. x?=w351:bool)
    n228 = Not(x=w358) -> (.not. x?=w350:bool)
    n229 = Not(x=w357) -> (.not. x?=w349:bool)
    n230 = Not(x=w356) -> (.not. x?=w348:bool)
    n231 = Not(x=w355) -> (.not. x?=w347:bool)
    n232 = local read "Iniciar"() -> (w417:bool)
    n233 = Build Array(w354, w353, w352, w351, w350, w349, w348, w347) -> (w336:bool[])
    n234 = Not(x=w417) -> (.not. x?=w416:bool)
    n235 = Not And(1:w417, 2:w419) -> (0:w423:bool)
    n236 = call "DAQ Assistant2"("data"=w336) -> ()  [unwired: 17 in, 2 out]
    n237 = Not And(1:w419, 2:w416) -> (0:w420:bool)
    n238 = feedback #3() -> (w421:bool)  [unwired: 1 in]
    n239 = Not And(1:w421, 2:w420) -> (0:w418:bool)
    "reset3" <- w418
    n240 = Not And(1:w423, 2:w418) -> (0:w422:bool)
    n241 = feedback-in #3(w422) -> ()
    n242 = local read "reset3"() -> (w403:bool)
    n243 = local read "q'"() -> (w375:bool)
    n244 = local read "q2'"() -> (w374:bool)
    n245 = case shown="True" w375 {
      frame False {
      }
      frame True {
        w707 = TRUE ("s")
        n246 = local read "reset"() -> (w710:bool)
        n247 = local read "Time"() -> (w712:dbl)
        n248 = call "Elapsed Time"("Time Target (s)"=w712, "Reset"=w710) -> ("Elapsed Time (s)"=w709:dbl, "Time has Elapsed"=→"Time has Elapsed":bool)  [unwired: 10 in, 6 out]
        "Tiempo" <- w709
        n249 = property on="Tiempo" class="DigNum (strict)"("Value"=w709) -> ()  [unwired: 2 in, 2 out]
        n250 = property on="Datapath" class="Bool (strict)"("Value"=w707) -> ()  [unwired: 2 in, 2 out]
        n251 = property on="Path1" class="Bool (strict)"("Value"=FALSE ("Boolean 19")) -> ()  [unwired: 2 in, 2 out]
        n252 = property on="Guardar" class="Bool (strict)"("Value"=w707) -> ()  [unwired: 2 in, 2 out]
        n253 = property on="Path2" class="Bool (strict)"("Value"=w707) -> ()  [unwired: 2 in, 2 out]
      }
    }
    n254 = case shown="True" "Iniciar" {
      tunnel: w403 -> [_ w715]
      frame False {
      }
      frame True {
        w713 = TRUE ("s")
        n255 = call "Elapsed Time3"("Reset"=w715) -> ("Elapsed Time (s)"=w714:dbl)  [unwired: 11 in, 7 out]
        "Tiempo" <- w714
        n256 = property on="Tiempo" class="DigNum (strict)"("Value"=w714) -> ()  [unwired: 2 in, 2 out]
        n257 = property on="Datapath" class="Bool (strict)"("Value"=w713) -> ()  [unwired: 2 in, 2 out]
        n258 = property on="Path1" class="Bool (strict)"("Value"=w713) -> ()  [unwired: 2 in, 2 out]
        n259 = property on="Guardar" class="Bool (strict)"("Value"=w713) -> ()  [unwired: 2 in, 2 out]
        n260 = property on="Path2" class="Bool (strict)"("Value"=w713) -> ()  [unwired: 2 in, 2 out]
      }
    }
    n261 = case shown="True" "Guardar Configuracion" {
      frame False {
      }
      frame True {
        w599 = "Offsets" ("section")
        w598 = TRUE ("use system decimal point (T)")
        w635 = TRUE ("write raw string? (F)")
        w632 = "Pendientes" ("section")
        w683 = "Nombres_Canales" ("section")
        n262 = call <vilib>:"Open Config Data.vi"("create file if necessary (T)"=TRUE, "configuration file path"=path "C:/Users/Zulueta/Documents/Pasantia/Configuracion") -> ("error out"=w671:errorcluster, "refnum"=w667:T3)  [unwired: 7 in, 1 out]
        n263 = local read "CH1"() -> (w684:string)
        n264 = call-poly <vilib>:"Write Key.vi"("write raw string? (F)"=w635, "section"=w683, "error in (no error)"=w671, "value"=w684, "key"="C1", "refnum"=w667) -> ("error out"=w672:errorcluster, "refnum out"=w668:T3)  [unwired: 3 in, 1 out]
        n265 = local read "CH2"() -> (w685:string)
        n266 = call-poly <vilib>:"Write Key.vi"("write raw string? (F)"=w635, "section"=w683, "error in (no error)"=w672, "value"=w685, "key"="C2", "refnum"=w668) -> ("error out"=w673:errorcluster, "refnum out"=w669:T3)  [unwired: 3 in, 1 out]
        n267 = local read "CH3"() -> (w686:string)
        n268 = call-poly <vilib>:"Write Key.vi"("write raw string? (F)"=w635, "section"=w683, "error in (no error)"=w673, "value"=w686, "key"="C3", "refnum"=w669) -> ("error out"=w674:errorcluster, "refnum out"=w670:T3)  [unwired: 3 in, 1 out]
        n269 = local read "CH4"() -> (w687:string)
        n270 = call-poly <vilib>:"Write Key.vi"("write raw string? (F)"=w635, "section"=w683, "error in (no error)"=w674, "value"=w687, "key"="C4", "refnum"=w670) -> ("error out"=w675:errorcluster, "refnum out"=w677:T3)  [unwired: 3 in, 1 out]
        n271 = local read "CH5"() -> (w688:string)
        n272 = call-poly <vilib>:"Write Key.vi"("write raw string? (F)"=w635, "section"=w683, "error in (no error)"=w675, "value"=w688, "key"="C5", "refnum"=w677) -> ("error out"=w676:errorcluster, "refnum out"=w678:T3)  [unwired: 3 in, 1 out]
        n273 = local read "CH6"() -> (w689:string)
        n274 = call-poly <vilib>:"Write Key.vi"("write raw string? (F)"=w635, "section"=w683, "error in (no error)"=w676, "value"=w689, "key"="C6", "refnum"=w678) -> ("error out"=w679:errorcluster, "refnum out"=w680:T3)  [unwired: 3 in, 1 out]
        n275 = local read "CH7"() -> (w690:string)
        n276 = call-poly <vilib>:"Write Key.vi"("write raw string? (F)"=w635, "section"=w683, "error in (no error)"=w679, "value"=w690, "key"="C7", "refnum"=w680) -> ("error out"=w682:errorcluster, "refnum out"=w681:T3)  [unwired: 3 in, 1 out]
        n277 = local read "CH8"() -> (w691:string)
        n278 = call-poly <vilib>:"Write Key.vi"("write raw string? (F)"=w635, "section"=w683, "error in (no error)"=w682, "value"=w691, "key"="C8", "refnum"=w681) -> ("error out"=w665:errorcluster, "refnum out"=w664:T3)  [unwired: 3 in, 1 out]
        n279 = local read "m1"() -> (w656:dbl)
        n280 = call-poly <vilib>:"Write Key.vi"("use system decimal point (T)"=w598, "section"=w632, "error in (no error)"=w665, "value"=w656, "key"="M1", "refnum"=w664) -> ("error out"=w662:errorcluster, "refnum out"=w663:T3)  [unwired: 3 in, 1 out]
        n281 = local read "m2"() -> (w655:dbl)
        n282 = call-poly <vilib>:"Write Key.vi"("use system decimal point (T)"=w598, "section"=w632, "error in (no error)"=w662, "value"=w655, "key"="M2", "refnum"=w663) -> ("error out"=w660:errorcluster, "refnum out"=w661:T3)  [unwired: 3 in, 1 out]
        n283 = local read "m3"() -> (w653:dbl)
        n284 = call-poly <vilib>:"Write Key.vi"("use system decimal point (T)"=w598, "section"=w632, "error in (no error)"=w660, "value"=w653, "key"="M3", "refnum"=w661) -> ("error out"=w658:errorcluster, "refnum out"=w659:T3)  [unwired: 3 in, 1 out]
        n285 = local read "m4"() -> (w651:dbl)
        n286 = call-poly <vilib>:"Write Key.vi"("use system decimal point (T)"=w598, "section"=w632, "error in (no error)"=w658, "value"=w651, "key"="M4", "refnum"=w659) -> ("error out"=w648:errorcluster, "refnum out"=w649:T3)  [unwired: 3 in, 1 out]
        n287 = local read "m5"() -> (w647:dbl)
        n288 = call-poly <vilib>:"Write Key.vi"("use system decimal point (T)"=w598, "section"=w632, "error in (no error)"=w648, "value"=w647, "key"="M5", "refnum"=w649) -> ("error out"=w642:errorcluster, "refnum out"=w643:T3)  [unwired: 3 in, 1 out]
        n289 = local read "m6"() -> (w645:dbl)
        n290 = call-poly <vilib>:"Write Key.vi"("use system decimal point (T)"=w598, "section"=w632, "error in (no error)"=w642, "value"=w645, "key"="M6", "refnum"=w643) -> ("error out"=w640:errorcluster, "refnum out"=w641:T3)  [unwired: 3 in, 1 out]
        n291 = local read "m7"() -> (w639:dbl)
        n292 = call-poly <vilib>:"Write Key.vi"("use system decimal point (T)"=w598, "section"=w632, "error in (no error)"=w640, "value"=w639, "key"="M7", "refnum"=w641) -> ("error out"=w636:errorcluster, "refnum out"=w637:T3)  [unwired: 3 in, 1 out]
        n293 = local read "m8"() -> (w634:dbl)
        n294 = call-poly <vilib>:"Write Key.vi"("use system decimal point (T)"=w598, "section"=w632, "error in (no error)"=w636, "value"=w634, "key"="M8", "refnum"=w637) -> ("error out"=w630:errorcluster, "refnum out"=w631:T3)  [unwired: 3 in, 1 out]
        n295 = local read "b1"() -> (w628:dbl)
        n296 = call-poly <vilib>:"Write Key.vi"("use system decimal point (T)"=w598, "section"=w599, "error in (no error)"=w630, "value"=w628, "key"="B1", "refnum"=w631) -> ("error out"=w626:errorcluster, "refnum out"=w627:T3)  [unwired: 3 in, 1 out]
        n297 = local read "b2"() -> (w624:dbl)
        n298 = call-poly <vilib>:"Write Key.vi"("use system decimal point (T)"=w598, "section"=w599, "error in (no error)"=w626, "value"=w624, "key"="B2", "refnum"=w627) -> ("error out"=w621:errorcluster, "refnum out"=w622:T3)  [unwired: 3 in, 1 out]
        n299 = local read "b3"() -> (w623:dbl)
        n300 = call-poly <vilib>:"Write Key.vi"("use system decimal point (T)"=w598, "section"=w599, "error in (no error)"=w621, "value"=w623, "key"="B3", "refnum"=w622) -> ("error out"=w618:errorcluster, "refnum out"=w619:T3)  [unwired: 3 in, 1 out]
        n301 = local read "b4"() -> (w617:dbl)
        n302 = call-poly <vilib>:"Write Key.vi"("use system decimal point (T)"=w598, "section"=w599, "error in (no error)"=w618, "value"=w617, "key"="B4", "refnum"=w619) -> ("error out"=w615:errorcluster, "refnum out"=w614:T3)  [unwired: 3 in, 1 out]
        n303 = local read "b5"() -> (w613:dbl)
        n304 = call-poly <vilib>:"Write Key.vi"("use system decimal point (T)"=w598, "section"=w599, "error in (no error)"=w615, "value"=w613, "key"="B5", "refnum"=w614) -> ("error out"=w611:errorcluster, "refnum out"=w610:T3)  [unwired: 3 in, 1 out]
        n305 = local read "b6"() -> (w609:dbl)
        n306 = call-poly <vilib>:"Write Key.vi"("use system decimal point (T)"=w598, "section"=w599, "error in (no error)"=w611, "value"=w609, "key"="B6", "refnum"=w610) -> ("error out"=w606:errorcluster, "refnum out"=w607:T3)  [unwired: 3 in, 1 out]
        n307 = local read "b7"() -> (w605:dbl)
        n308 = call-poly <vilib>:"Write Key.vi"("use system decimal point (T)"=w598, "section"=w599, "error in (no error)"=w606, "value"=w605, "key"="B7", "refnum"=w607) -> ("error out"=w602:errorcluster, "refnum out"=w603:T3)  [unwired: 3 in, 1 out]
        n309 = local read "b8"() -> (w601:dbl)
        n310 = call-poly <vilib>:"Write Key.vi"("use system decimal point (T)"=w598, "section"=w599, "error in (no error)"=w602, "value"=w601, "key"="B8", "refnum"=w603) -> ("error out"=w596:errorcluster, "refnum out"=w597:T3)  [unwired: 3 in, 1 out]
        n311 = call <vilib>:"Close Config Data.vi"("error in (no error)"=w596, "refnum"=w597) -> ()  [unwired: 8 in, 2 out]
      }
    }
    n312 = case shown="True" w374 {
      frame False {
      }
      frame True {
        w702 = FALSE ("s")
        n313 = local read "reset2"() -> (w704:bool)
        n314 = local read "Time"() -> (w706:dbl)
        n315 = call "Elapsed Time2"("Time Target (s)"=w706, "Reset"=w704) -> ("Elapsed Time (s)"=w701:dbl, "Time has Elapsed"=→"Time has Elapsed 2":bool)  [unwired: 10 in, 6 out]
        "Tiempo" <- w701
        n316 = property on="Tiempo" class="DigNum (strict)"("Value"=w701) -> ()  [unwired: 2 in, 2 out]
        n317 = property on="Datapath" class="Bool (strict)"("Value"=w702) -> ()  [unwired: 2 in, 2 out]
        n318 = property on="Path2" class="Bool (strict)"("Value"=w702) -> ()  [unwired: 2 in, 2 out]
        n319 = property on="Guardar" class="Bool (strict)"("Value"=TRUE ("y")) -> ()  [unwired: 2 in, 2 out]
      }
    }
    n320 = Or(x=w375, y=w374) -> (x .or. y?=w376:bool)
    n321 = Or(x="Iniciar", y=w376) -> (x .or. y?=w384:bool)
    n322 = case shown="False" w384 {
      frame False {
        n323 = property on="index" class="DigNum (strict)"() -> ("Value"=w451:i32)  [unwired: 2 in, 2 out]
        n324 = property on="index 3" class="DigNum (strict)"("Value"=w451) -> ()  [unwired: 2 in, 2 out]
      }
      frame True {
      }
    }
    n325 = Not(x=w384) -> (.not. x?=w405:bool)
    n326 = And(x=w405, y="Guardar") -> (x .and. y?=w404:bool)
    n327 = Select(t=w383, s="Path1", f=w382) -> (s? t:f=w380:refnum<k34>)
    n328 = Select(t=w380, s="Path2", f=w373) -> (s? t:f=w379:refnum<k34>)
    n329 = case shown="True" w404 {
      tunnel: w399 -> [_ w585]
      tunnel: w398 -> [_ w584]
      tunnel: w397 -> [_ w583]
      tunnel: w396 -> [_ w582]
      tunnel: w390 -> [_ w581]
      tunnel: w395 -> [_ w580]
      tunnel: w389 -> [_ w579]
      tunnel: w394 -> [_ w578]
      tunnel: w388 -> [_ w577]
      tunnel: w393 -> [_ w576]
      tunnel: w387 -> [_ w575]
      tunnel: w392 -> [_ w574]
      tunnel: w386 -> [_ w573]
      tunnel: w391 -> [_ w572]
      tunnel: w400 -> [_ w571]
      tunnel: w379 -> [_ w557]
      tunnel: w346 -> [_ w519]
      frame False {
      }
      frame True {
        w452 = enum16{"Sample", "Population"}."Population" ("Weighting (Sample)")
        w570 = TRUE ("return elements? (F)")
        n330 = property on="Tasa de Adquisicion" class="DigNum (strict)"() -> ("Value"=w594:dbl)  [unwired: 2 in, 2 out]
        n331 = Multiply(x="Tiempo", y=w594) -> (x*y=w593:dbl)
        n332 = Round Toward -Infinity(1:w593) -> (0:w561:dbl)
        n333 = Get Queue Status(queue=w519, return elements? (F)=w570) -> (elements=w595:dbl[])  [unwired: 1 in, 7 out]
        n334 = Get Queue Status(queue=w585, return elements? (F)=w570) -> (elements=w592:dbl[])  [unwired: 1 in, 7 out]
        n335 = Get Queue Status(queue=w584, return elements? (F)=w570) -> (elements=w591:dbl[])  [unwired: 1 in, 7 out]
        n336 = Get Queue Status(queue=w583, return elements? (F)=w570) -> (elements=w590:dbl[])  [unwired: 1 in, 7 out]
        n337 = Get Queue Status(queue=w582, return elements? (F)=w570) -> (elements=w589:dbl[])  [unwired: 1 in, 7 out]
        n338 = Get Queue Status(queue=w580, return elements? (F)=w570) -> (elements=w587:dbl[])  [unwired: 1 in, 7 out]
        n339 = Get Queue Status(queue=w579, return elements? (F)=w570) -> (elements=w586:dbl[])  [unwired: 1 in, 7 out]
        n340 = Get Queue Status(queue=w578, return elements? (F)=w570) -> (elements=w569:dbl[])  [unwired: 1 in, 7 out]
        n341 = Get Queue Status(queue=w577, return elements? (F)=w570) -> (elements=w568:dbl[])  [unwired: 1 in, 7 out]
        n342 = Get Queue Status(queue=w576, return elements? (F)=w570) -> (elements=w567:dbl[])  [unwired: 1 in, 7 out]
        n343 = Get Queue Status(queue=w575, return elements? (F)=w570) -> (elements=w566:dbl[])  [unwired: 1 in, 7 out]
        n344 = Get Queue Status(queue=w574, return elements? (F)=w570) -> (elements=w565:dbl[])  [unwired: 1 in, 7 out]
        n345 = Get Queue Status(queue=w573, return elements? (F)=w570) -> (elements=w564:dbl[])  [unwired: 1 in, 7 out]
        n346 = Get Queue Status(queue=w572, return elements? (F)=w570) -> (elements=w563:dbl[])  [unwired: 1 in, 7 out]
        n347 = Get Queue Status(queue=w571, return elements? (F)=w570) -> (elements=w562:dbl[])  [unwired: 1 in, 7 out]
        n348 = Get Queue Status(queue=w581, return elements? (F)=w570) -> (elements=w588:dbl[])  [unwired: 1 in, 7 out]
        n349 = Array Subset(array=w595, index="index 3", length=w561) -> (w517:dbl[])
        n350 = Array Subset(array=w592, index="index 3", length=w561) -> (w527:dbl[])
        n351 = Array Subset(array=w591, index="index 3", length=w561) -> (w529:dbl[])
        n352 = Array Subset(array=w590, index="index 3", length=w561) -> (w531:dbl[])
        n353 = Array Subset(array=w589, index="index 3", length=w561) -> (w533:dbl[])
        n354 = Array Subset(array=w588, index="index 3", length=w561) -> (w535:dbl[])
        n355 = Array Subset(array=w587, index="index 3", length=w561) -> (w537:dbl[])
        n356 = Array Subset(array=w586, index="index 3", length=w561) -> (w539:dbl[])
        n357 = Array Subset(array=w569, index="index 3", length=w561) -> (w541:dbl[])
        n358 = Array Subset(array=w568, index="index 3", length=w561) -> (w543:dbl[])
        n359 = Array Subset(array=w567, index="index 3", length=w561) -> (w545:dbl[])
        n360 = Array Subset(array=w566, index="index 3", length=w561) -> (w547:dbl[])
        n361 = Array Subset(array=w565, index="index 3", length=w561) -> (w549:dbl[])
        n362 = Array Subset(array=w564, index="index 3", length=w561) -> (w551:dbl[])
        n363 = Array Subset(array=w563, index="index 3", length=w561) -> (w553:dbl[])
        n364 = Array Subset(array=w562, index="index 3", length=w561) -> (w555:dbl[])
        n365 = call <vilib>:"Std Deviation and Variance.vi"("X"=w517, "Weighting (Sample)"=w452) -> ("mean"=w516:dbl, "standard deviation"=w515:dbl)  [unwired: 1 out]
        n366 = call <vilib>:"Std Deviation and Variance.vi"("X"=w527, "Weighting (Sample)"=w452) -> ("mean"=w512:dbl, "standard deviation"=w511:dbl)  [unwired: 1 out]
        n367 = call <vilib>:"Std Deviation and Variance.vi"("X"=w529, "Weighting (Sample)"=w452) -> ("mean"=w508:dbl, "standard deviation"=w507:dbl)  [unwired: 1 out]
        n368 = call <vilib>:"Std Deviation and Variance.vi"("X"=w531, "Weighting (Sample)"=w452) -> ("mean"=w504:dbl, "standard deviation"=w503:dbl)  [unwired: 1 out]
        n369 = call <vilib>:"Std Deviation and Variance.vi"("X"=w533, "Weighting (Sample)"=w452) -> ("mean"=w500:dbl, "standard deviation"=w499:dbl)  [unwired: 1 out]
        n370 = call <vilib>:"Std Deviation and Variance.vi"("X"=w535, "Weighting (Sample)"=w452) -> ("mean"=w495:dbl, "standard deviation"=w491:dbl)  [unwired: 1 out]
        n371 = call <vilib>:"Std Deviation and Variance.vi"("X"=w537, "Weighting (Sample)"=w452) -> ("mean"=w496:dbl, "standard deviation"=w490:dbl)  [unwired: 1 out]
        n372 = call <vilib>:"Std Deviation and Variance.vi"("X"=w539, "Weighting (Sample)"=w452) -> ("mean"=w494:dbl, "standard deviation"=w489:dbl)  [unwired: 1 out]
        n373 = call <vilib>:"Std Deviation and Variance.vi"("X"=w541, "Weighting (Sample)"=w452) -> ("mean"=w493:dbl, "standard deviation"=w488:dbl)  [unwired: 1 out]
        n374 = call <vilib>:"Std Deviation and Variance.vi"("X"=w543, "Weighting (Sample)"=w452) -> ("mean"=w492:dbl, "standard deviation"=w487:dbl)  [unwired: 1 out]
        n375 = call <vilib>:"Std Deviation and Variance.vi"("X"=w545, "Weighting (Sample)"=w452) -> ("mean"=w476:dbl, "standard deviation"=w465:dbl)  [unwired: 1 out]
        n376 = call <vilib>:"Std Deviation and Variance.vi"("X"=w547, "Weighting (Sample)"=w452) -> ("mean"=w475:dbl, "standard deviation"=w466:dbl)  [unwired: 1 out]
        n377 = call <vilib>:"Std Deviation and Variance.vi"("X"=w549, "Weighting (Sample)"=w452) -> ("mean"=w474:dbl, "standard deviation"=w467:dbl)  [unwired: 1 out]
        n378 = call <vilib>:"Std Deviation and Variance.vi"("X"=w551, "Weighting (Sample)"=w452) -> ("mean"=w473:dbl, "standard deviation"=w468:dbl)  [unwired: 1 out]
        n379 = call <vilib>:"Std Deviation and Variance.vi"("X"=w553, "Weighting (Sample)"=w452) -> ("mean"=w472:dbl, "standard deviation"=w469:dbl)  [unwired: 1 out]
        n380 = call <vilib>:"Std Deviation and Variance.vi"("X"=w555, "Weighting (Sample)"=w452) -> ("mean"=w471:dbl, "standard deviation"=w470:dbl)  [unwired: 1 out]
        n381 = call "Convert to Dynamic Data16"("Array"=w517) -> ("Dynamic Data Type"=w525:dynamicdata)  [unwired: 3 in]
        n382 = call "Convert to Dynamic Data15"("Array"=w527) -> ("Dynamic Data Type"=w526:dynamicdata)  [unwired: 3 in]
        n383 = call "Convert to Dynamic Data14"("Array"=w529) -> ("Dynamic Data Type"=w528:dynamicdata)  [unwired: 3 in]
        n384 = call "Convert to Dynamic Data13"("Array"=w531) -> ("Dynamic Data Type"=w530:dynamicdata)  [unwired: 3 in]
        n385 = call "Convert to Dynamic Data12"("Array"=w533) -> ("Dynamic Data Type"=w532:dynamicdata)  [unwired: 3 in]
        n386 = call "Convert to Dynamic Data11"("Array"=w535) -> ("Dynamic Data Type"=w534:dynamicdata)  [unwired: 3 in]
        n387 = call "Convert to Dynamic Data10"("Array"=w537) -> ("Dynamic Data Type"=w536:dynamicdata)  [unwired: 3 in]
        n388 = call "Convert to Dynamic Data9"("Array"=w539) -> ("Dynamic Data Type"=w538:dynamicdata)  [unwired: 3 in]
        n389 = call "Convert to Dynamic Data8"("Array"=w541) -> ("Dynamic Data Type"=w540:dynamicdata)  [unwired: 3 in]
        n390 = call "Convert to Dynamic Data7"("Array"=w543) -> ("Dynamic Data Type"=w542:dynamicdata)  [unwired: 3 in]
        n391 = call "Convert to Dynamic Data6"("Array"=w545) -> ("Dynamic Data Type"=w544:dynamicdata)  [unwired: 3 in]
        n392 = call "Convert to Dynamic Data5"("Array"=w547) -> ("Dynamic Data Type"=w546:dynamicdata)  [unwired: 3 in]
        n393 = call "Convert to Dynamic Data4"("Array"=w549) -> ("Dynamic Data Type"=w548:dynamicdata)  [unwired: 3 in]
        n394 = call "Convert to Dynamic Data3"("Array"=w551) -> ("Dynamic Data Type"=w550:dynamicdata)  [unwired: 3 in]
        n395 = call "Convert to Dynamic Data2"("Array"=w553) -> ("Dynamic Data Type"=w552:dynamicdata)  [unwired: 3 in]
        n396 = call "Convert to Dynamic Data"("Array"=w555) -> ("Dynamic Data Type"=w554:dynamicdata)  [unwired: 3 in]
        n397 = Build Array(w516, w515) -> (w514:dbl[])
        n398 = Build Array(w512, w511) -> (w510:dbl[])
        n399 = Build Array(w508, w507) -> (w506:dbl[])
        n400 = Build Array(w504, w503) -> (w502:dbl[])
        n401 = Build Array(w500, w499) -> (w498:dbl[])
        n402 = Build Array(w495, w491) -> (w486:dbl[])
        n403 = Build Array(w496, w490) -> (w484:dbl[])
        n404 = Build Array(w494, w489) -> (w482:dbl[])
        n405 = Build Array(w493, w488) -> (w480:dbl[])
        n406 = Build Array(w492, w487) -> (w478:dbl[])
        n407 = Build Array(w476, w465) -> (w464:dbl[])
        n408 = Build Array(w475, w466) -> (w462:dbl[])
        n409 = Build Array(w474, w467) -> (w460:dbl[])
        n410 = Build Array(w473, w468) -> (w458:dbl[])
        n411 = Build Array(w472, w469) -> (w456:dbl[])
        n412 = Build Array(w471, w470) -> (w454:dbl[])
        n413 = Merge Signals(w525, w526, w528, w530, w532, w534, w536, w538, w540, w542, w544, w546, w548, w550, w552, w554) -> (w524:dynamicdata)
        n414 = local read "appended array"() -> (w559:string[])
        n415 = call "Convert to Dynamic Data17"("Array"=w514) -> ("Dynamic Data Type"=w513:dynamicdata)  [unwired: 3 in]
        n416 = call "Convert to Dynamic Data18"("Array"=w510) -> ("Dynamic Data Type"=w509:dynamicdata)  [unwired: 3 in]
        n417 = call "Convert to Dynamic Data19"("Array"=w506) -> ("Dynamic Data Type"=w505:dynamicdata)  [unwired: 3 in]
        n418 = call "Convert to Dynamic Data20"("Array"=w502) -> ("Dynamic Data Type"=w501:dynamicdata)  [unwired: 3 in]
        n419 = call "Convert to Dynamic Data21"("Array"=w498) -> ("Dynamic Data Type"=w497:dynamicdata)  [unwired: 3 in]
        n420 = call "Convert to Dynamic Data22"("Array"=w486) -> ("Dynamic Data Type"=w485:dynamicdata)  [unwired: 3 in]
        n421 = call "Convert to Dynamic Data23"("Array"=w484) -> ("Dynamic Data Type"=w483:dynamicdata)  [unwired: 3 in]
        n422 = call "Convert to Dynamic Data24"("Array"=w482) -> ("Dynamic Data Type"=w481:dynamicdata)  [unwired: 3 in]
        n423 = call "Convert to Dynamic Data25"("Array"=w480) -> ("Dynamic Data Type"=w479:dynamicdata)  [unwired: 3 in]
        n424 = call "Convert to Dynamic Data26"("Array"=w478) -> ("Dynamic Data Type"=w477:dynamicdata)  [unwired: 3 in]
        n425 = call "Convert to Dynamic Data27"("Array"=w464) -> ("Dynamic Data Type"=w463:dynamicdata)  [unwired: 3 in]
        n426 = call "Convert to Dynamic Data28"("Array"=w462) -> ("Dynamic Data Type"=w461:dynamicdata)  [unwired: 3 in]
        n427 = call "Convert to Dynamic Data29"("Array"=w460) -> ("Dynamic Data Type"=w459:dynamicdata)  [unwired: 3 in]
        n428 = call "Convert to Dynamic Data30"("Array"=w458) -> ("Dynamic Data Type"=w457:dynamicdata)  [unwired: 3 in]
        n429 = call "Convert to Dynamic Data31"("Array"=w456) -> ("Dynamic Data Type"=w455:dynamicdata)  [unwired: 3 in]
        n430 = call "Convert to Dynamic Data32"("Array"=w454) -> ("Dynamic Data Type"=w453:dynamicdata)  [unwired: 3 in]
        n431 = Merge Signals(w513, w509, w505, w501, w497, w485, w483, w481, w479, w477, w463, w461, w459, w457, w455, w453) -> (w523:dynamicdata)
        n432 = Select(t=w524, s="Datapath", f=w523) -> (s? t:f=w522:dynamicdata)
        n433 = TDMS Write(0:w557, 1:enum16{"decimated", "interleaved"}."decimated" ("data layout (0:decimated)"), 5:"Mediciones USB-6009" ("group name in (Untitled)"), 7:w559, 9:w522) -> ()  [unwired: 1 in, 4 out]
        n434 = property on="Guardar" class="Bool (strict)"("Value"=FALSE ("Boolean 18")) -> ()  [unwired: 2 in, 2 out]
      }
    }
    n435 = property on="Boolean 10" class="Bool (strict)"() -> ("Value"=w337:bool)  [unwired: 2 in, 2 out]
    "CH1" <- "CH1"
    "CH2" <- "CH2 2"
    "CH3" <- "CH3"
    "CH4" <- "CH4 2"
    "CH5" <- "CH5"
    "CH6" <- "CH6"
    "CH7" <- "CH7"
    "CH8" <- "CH8"
    "Boolean 9" <- "Iniciar"
    "CH1" <- "CH1"
    "CH2" <- "CH2 2"
    "CH3" <- "CH3"
    "CH4" <- "CH4 2"
    "CH5" <- "CH5"
    "CH6" <- "CH6"
    "CH7" <- "CH7"
    "CH8" <- "CH8"
  }
